vi "Get Image.vi"(8 "error in (no error)":errorcluster, 11 "Bobcat 640 in":refnum<class "Bobcat 640.lvclass">) -> (0 "error out":errorcluster, 3 "Bobcat 640 out":refnum<class "Bobcat 640.lvclass">)   [LabVIEW 2018, in "Bobcat 640.lvlib" / "Bobcat 640.lvclass"]
uses:
  Bobcat 640.lvclass
  PPLs/Camera/Parent/Camera.lvlibp/1abvi3w/vi.lib/vision/Image Controls.llb/IMAQ Image.ctl
  PPLs/Camera/Parent/Camera.lvlibp/Camera.lvclass
  C:/AME Test Engineering/LabVIEW/PPLs/Camera/Parent/Camera.lvlibp/Camera.lvclass
  PPLs/Camera/Parent/Camera.lvlibp
panel:
  out "Image":T1
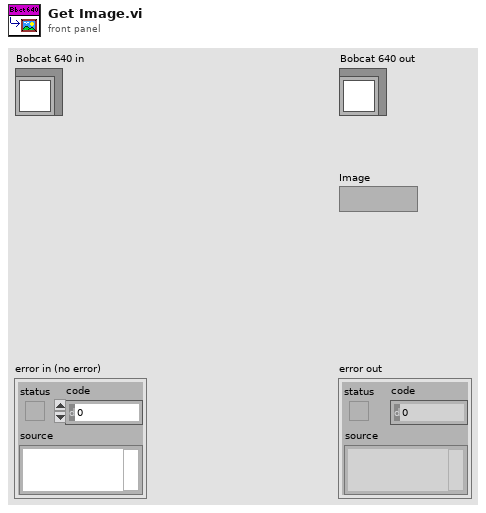
[diagram p1: front panel]
types:
  T1 = typedef "Camera.lvlibp/IMAQ Image.ctl" = refnum<image>
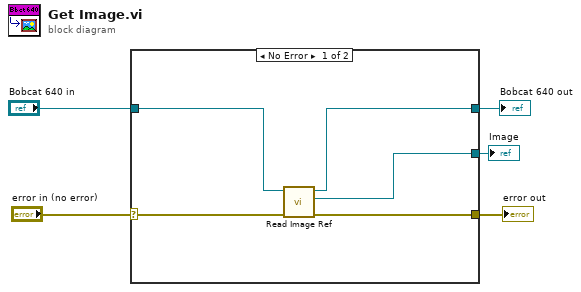
[diagram p0: block diagram]
diagram:
  n1 = case shown="No Error" "error in (no error)" {
    selector: "error in (no error)" -> [w9 w12]
    tunnel: [w8 w12] -> w4
    tunnel: [w6 w11] -> w2
    tunnel: "Bobcat 640 in" -> [w10 w11]
    tunnel: [w7 _] -> w1
    frame No Error {
      n2 = call "Read Image Ref.vi"("error in (no error)"=w9, "Camera in"=w10) -> ("error out"=w8:errorcluster, "Image"=w7:T1, "Camera out"=w6:refnum<class "Bobcat 640.lvclass">)  [unwired: 7 in]
    }
    frame Error {
    }
  }
  "error out" <- w4
  "Bobcat 640 out" <- w2
  "Image" <- w1
